vi "PC_save_output_settings_to_csv.vi"(8 "error in (no error)":errorcluster, 9 "settings":T1, 10 "Save?":bool, 11 "File Parameters":cluster{"Path":path, "Recording Name":string}={"Path"=path "D:/data/Lucas/20210707_lucas_test_saving", "Recording Name"=""}) -> (0 "error out":errorcluster, 3 "file path out":string)   [LabVIEW 2020]
uses:
  output_headers.ctl
  output_settings.ctl
  <vilib>/Utility/file.llb/Write Delimited Spreadsheet (string).vi
panel:
  out "Array":string[](array[string])
  in  "Headers":T2=["timestamp", "ac_freq", "ac_volt", "mod_waveform", "mod_freq", "mod_depth", "dio0", "dio1", "dio2", "dio3"]
  in  "Seconds In File":dbl
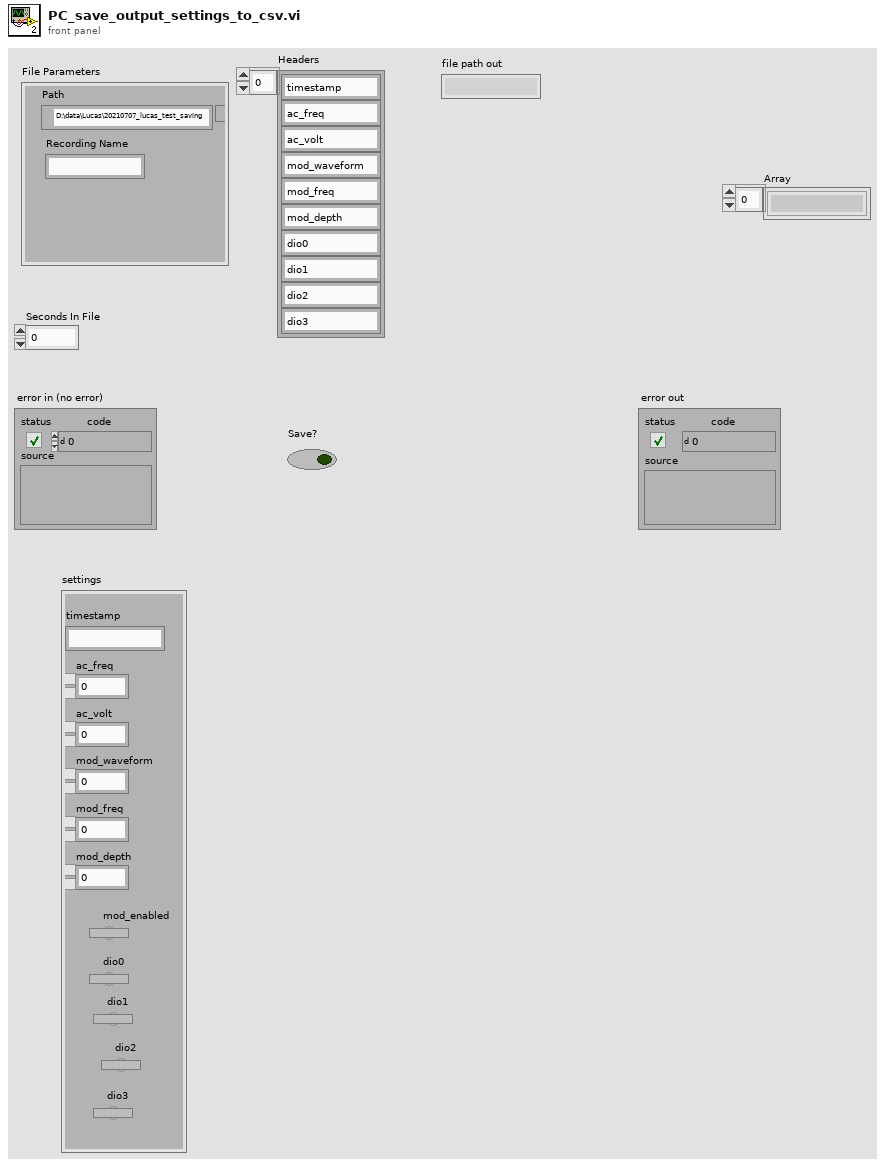
[diagram p1: front panel]
types:
  T1 = typedef "output_settings.ctl" = cluster{"timestamp":string, "ac_freq":dbl, "ac_volt":dbl, "mod_waveform":dbl, "mod_freq":dbl, "mod_depth":dbl, "dio1":bool, "dio2":bool, "dio3":bool, "dio0":bool, "mod_enabled":bool}
  T2 = typedef "output_headers.ctl" = string[]
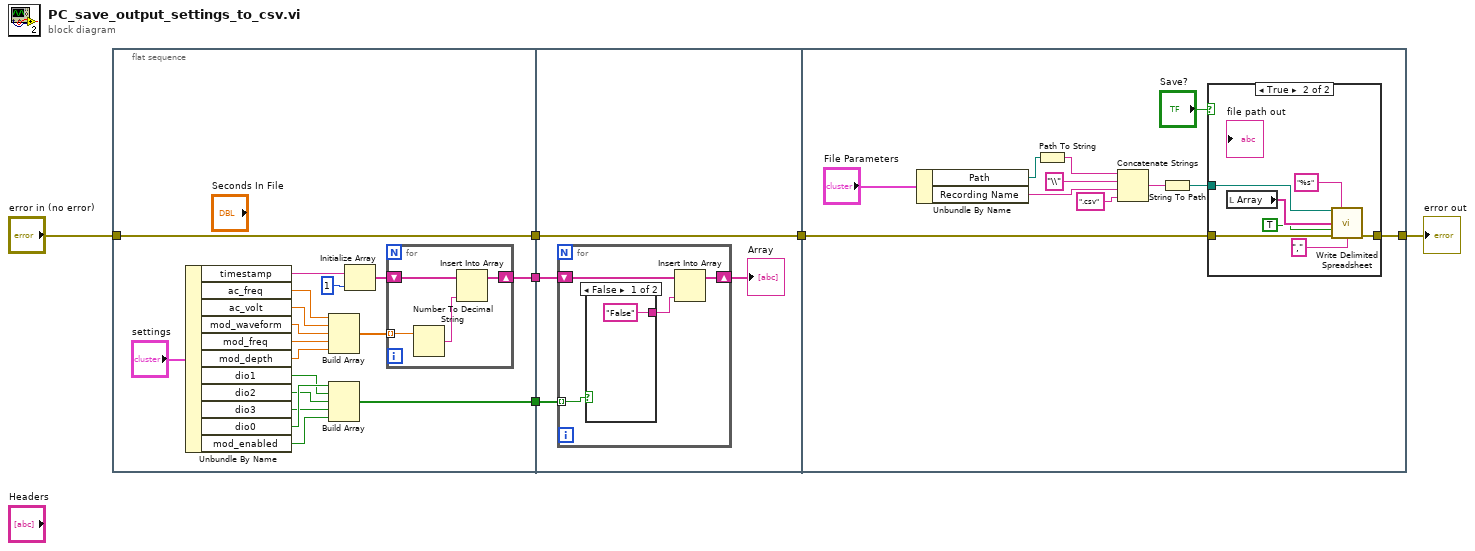
[diagram p0: block diagram]
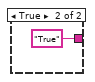
[diagram p2: hidden frame]
diagram:
  n1 = flat-sequence {
    tunnel: [w24] -> w4
    tunnel: "error in (no error)" -> [w24]
    tunnel: [w23] -> w2
    tunnel: [w20] -> w1
    tunnel: w4 -> [w32]
    tunnel: [w32] -> w3
    tunnel: w2 -> [w29]
    tunnel: w1 -> [w31]
    tunnel: w3 -> [w49]
    tunnel: [w47] -> w5
    frame #0 {
      n2 = Unbundle By Name("settings") -> ("timestamp"=w17:string, "ac_freq"=w16:dbl, "ac_volt"=w15:dbl, "mod_waveform"=w14:dbl, "mod_freq"=w13:dbl, "mod_depth"=w7:dbl, "dio1"=w11:bool, "dio2"=w10:bool, "dio3"=w9:bool, "dio0"=w12:bool, "mod_enabled"=w8:bool)
      n3 = Build Array(w16, w15, w14, w13, w7) -> (w22:dbl[])
      n4 = Build Array(w12, w11, w10, w9, w8) -> (w23:bool[])
      n5 = Initialize Array(w17, 1 ("dimension size")) -> (w21:string[])
      n6 = for {
        tunnel: w22 -> [w28] mode=indexing
        shift-right: [w27] -> w20
        shift-left: w21 -> [w26]
        n7 = Number To Decimal String(number=w28) -> (decimal integer string=w25:string)  [unwired: 1 in]
        n8 = Insert Into Array(array=w26, new element=w25) -> (w27:string[])  [unwired: 1 in]
      }
    }
    frame #1 {
      n9 = for {
        tunnel: w29 -> [w35] mode=indexing
        shift-right: [w33] -> w30
        shift-left: w31 -> [w34]
        n10 = case shown="False" w35 {
          tunnel: ["False" "True"] -> w36
          frame False {
          }
          frame True {
          }
        }
        n11 = Insert Into Array(array=w34, new element=w36) -> (w33:string[])  [unwired: 1 in]
      }
      "Array" <- w30
    }
    frame #2 {
      n12 = Unbundle By Name("File Parameters") -> ("Path"=w43:path, "Recording Name"=w46:string)
      n13 = Path To String(path=w43) -> (string=w44:string)
      n14 = Concatenate Strings(w44, "\\", w46, ".csv") -> (w45:string)
      n15 = String To Path(string=w45) -> (path=w39:path)
      n16 = case shown="True" "Save?" {
        tunnel: w49 -> [w50 w56]
        tunnel: w39 -> [_ w57]
        tunnel: [w50 w54] -> w47
        frame False {
        }
        frame True {
          n17 = local read "Array"() -> (w53:string[])
          n18 = call-poly <vilib>:"Write Delimited Spreadsheet.vi"("file path (dialog if empty)"=w57, "format (%s)"="%s", "1D data"=w53, "append to file? (new file:F)"=TRUE, "error in (no error)"=w56, "delimiter (\\t)"="," ("delimiter (\\t)")) -> ("error out"=w54:errorcluster)  [unwired: 8 in, 1 out]
        }
      }
    }
  }
  "error out" <- w5
